vi "TP_FGV_Log.vi"(7 "Enum":T1(ring)=enum."GetValue", 8 "error in":errorcluster, 10 "Log Path":path, 11 "log":string) -> (0 "error out":errorcluster)   [LabVIEW 2012]
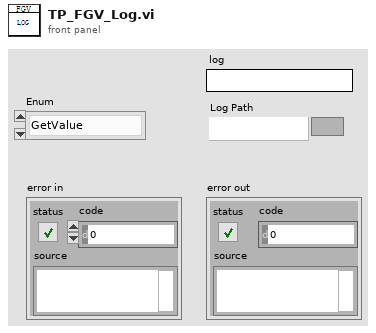
[diagram p1: front panel]
types:
  T1 = enum16{"Init", "GetValue", "SetValue", "Destory", "ErrLog"}
  T2 = enum16{"open", "replace", "create", "open or create", "replace or create", "replace or create with confirmation"}
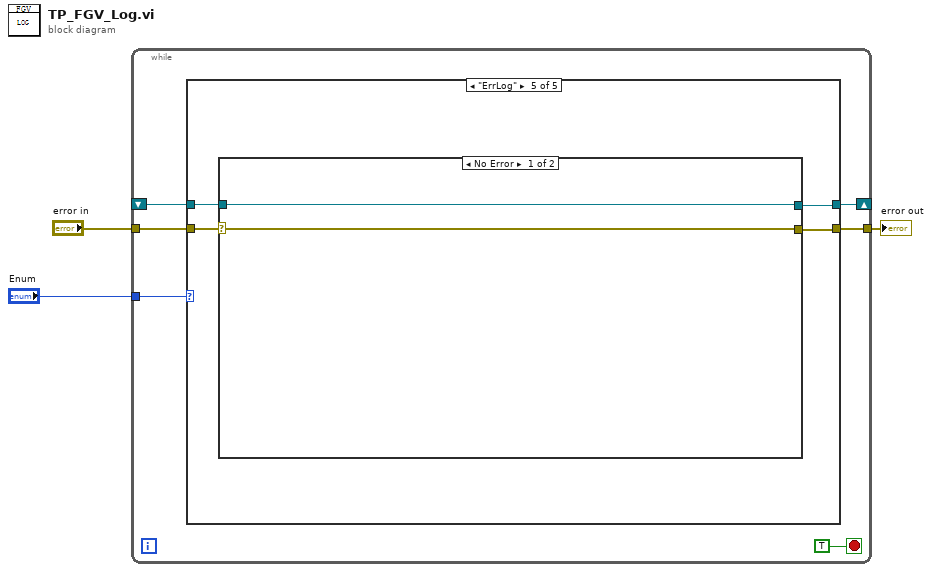
[diagram p0: block diagram]
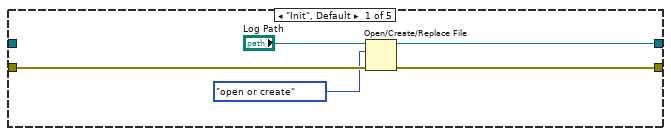
[diagram p2: hidden frame]
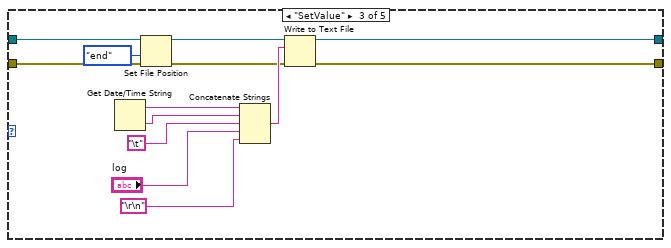
[diagram p4: hidden frame]
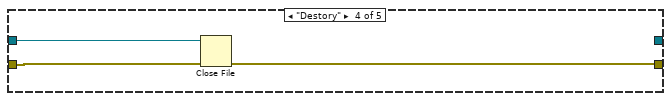
[diagram p5: hidden frame]
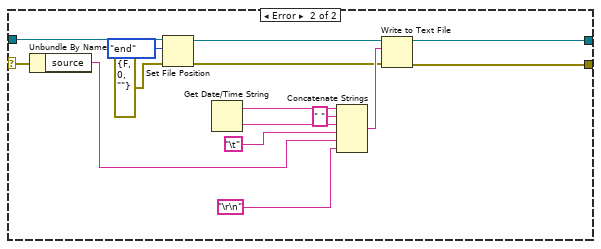
[diagram p6: hidden frame]
diagram:
  n1 = while {
    tunnel: "Enum" -> [w9]
    shift-right: [w7] -> _
    shift-left: _ -> [w8]
    tunnel: [w6] -> w2
    tunnel: "error in" -> [w5]
    stop <- TRUE stop-if-true
    n2 = case shown="\"ErrLog\"" w9 {
      tunnel: w8 -> [_ w16 w19 w30 w34]
      tunnel: [w14 w16 w28 _ w36] -> w7
      tunnel: [w13 w15 w29 w31 w35] -> w6
      tunnel: w5 -> [w12 w15 w21 w32 w33]
      frame "Init", Default {
        n3 = Open/Create/Replace File(file path (use dialog)="Log Path", error in=w12, operation (0:open)=T2."open or create") -> (refnum out=w14:refnum<file>, error out=w13:errorcluster)  [unwired: 3 in, 1 out]
      }
      frame "GetValue" {
      }
      frame "SetValue" {
        n4 = Get Date/Time String() -> (date string=w27:string, time string=w26:string)  [unwired: 3 in]
        n5 = Set File Position(refnum=w19, from (0:start)=enum16{"start", "end", "current"}."end", error in=w21) -> (refnum out=w18:refnum<file>, error out=w20:errorcluster)  [unwired: 1 in]
        n6 = Concatenate Strings(w27, w26, "\t", "log", "\r\n") -> (w22:string)
        n7 = Write to Text File(file (use dialog)=w18, text=w22, error in=w20) -> (refnum out=w28:refnum<file>, error out=w29:errorcluster)  [unwired: 1 in, 1 out]
      }
      frame "Destory" {
        n8 = Close File(refnum=w30, error in=w32) -> (error out=w31:errorcluster)  [unwired: 1 out]
      }
      frame "ErrLog" {
        n9 = case shown="No Error" w33 {
          selector: w33 -> [w37 w41]
          tunnel: [w38 w49] -> w36
          tunnel: [w37 w47] -> w35
          tunnel: w34 -> [w38 w46]
          frame No Error {
          }
          frame Error {
            n10 = Unbundle By Name(w41) -> ("source"=w48:string)
            n11 = Set File Position(refnum=w46, from (0:start)=enum16{"start", "end", "current"}."end", error in=errorcluster {"status"=FALSE, "code"=0, "source"=""}) -> (refnum out=w42:refnum<file>, error out=w44:errorcluster)  [unwired: 1 in]
            n12 = Get Date/Time String() -> (date string=w40:string, time string=w53:string)  [unwired: 3 in]
            n13 = Concatenate Strings(w40, " " ("string"), w53, "\t", w48, "\r\n") -> (w50:string)
            n14 = Write to Text File(file (use dialog)=w42, text=w50, error in=w44) -> (refnum out=w49:refnum<file>, error out=w47:errorcluster)  [unwired: 1 in, 1 out]
          }
        }
      }
    }
  }
  "error out" <- w2
